vi "New TCP Socket from Refnum.vi"(8 "error in (no error)":errorcluster, 11 "TCP Network Connection Refnum":refnum<k5>) -> (0 "error out":errorcluster, 3 "VISA TCP out":refnum<class "VISA TCP.lvclass">)   [LabVIEW 2021, in "Sockets.lvlib" / "VISA TCP.lvclass"]
doc: "Upgrades an existing VISA TCP refnum to a VISA TCP Socket.\nWebSockets 2.0.1.40\nSam Sharp - MediaMongrels Ltd\nCopyright (c) 2019, MediaMongrels Ltd"
uses:
  VISA TCP.lvclass
  VISA TCP.lvclass/VISA TCP.ctl
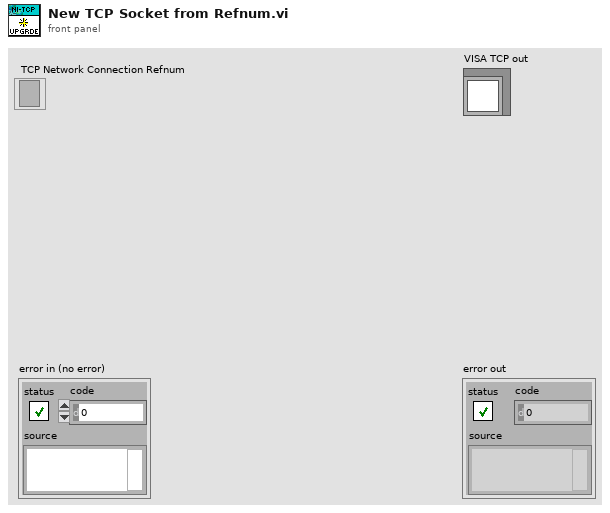
[diagram p1: front panel]
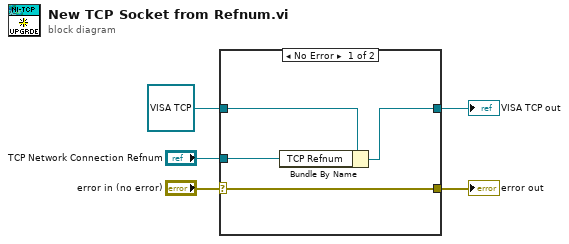
[diagram p0: block diagram]
diagram:
  n1 = case shown="No Error" "error in (no error)" {
    selector: "error in (no error)" -> [w9 w11]
    tunnel: [w9 w11] -> w4
    tunnel: [w7 w10] -> w3
    tunnel: refnum<class "VISA TCP.lvclass"> refnum ("VISA TCP in") -> [w8 w10]
    tunnel: "TCP Network Connection Refnum" -> [w6 _]
    frame No Error {
      n2 = Bundle By Name(cluster=w8, "TCP Refnum"=w6) -> (w7:refnum<class "VISA TCP.lvclass">)
    }
    frame Error {
    }
  }
  "error out" <- w4
  "VISA TCP out" <- w3
